vi "Discover Devices.vi"(8 "error in (no error)":errorcluster, 11 "Tree ref in":refnum<vi>) -> (0 "error out":errorcluster)   [LabVIEW 2022 SP3]
doc: "This example demonstrated how to create an openDAQ instance and detect devices.\nThen it goes through all detected devices and displays their name and manufacturer."
uses:
  <instrlib>/openDAQ/Public/Classes/IInstance/IInstance.lvclass
  C:/Program Files (x86)/National Instruments/LabVIEW 2022/instr.lib/openDAQ/Public/Classes/IDevice/IDevice.lvclass
  <instrlib>/openDAQ/Public/Classes/IInstanceBuilder/IInstanceBuilder.lvclass
  <instrlib>/openDAQ/Public/Classes/IDeviceInfo/IDeviceInfo.lvclass
  <instrlib>/openDAQ/Public/Classes/IDevice/IDevice.lvclass
panel:
  in  "MCL:available Devices":i32(listbox)
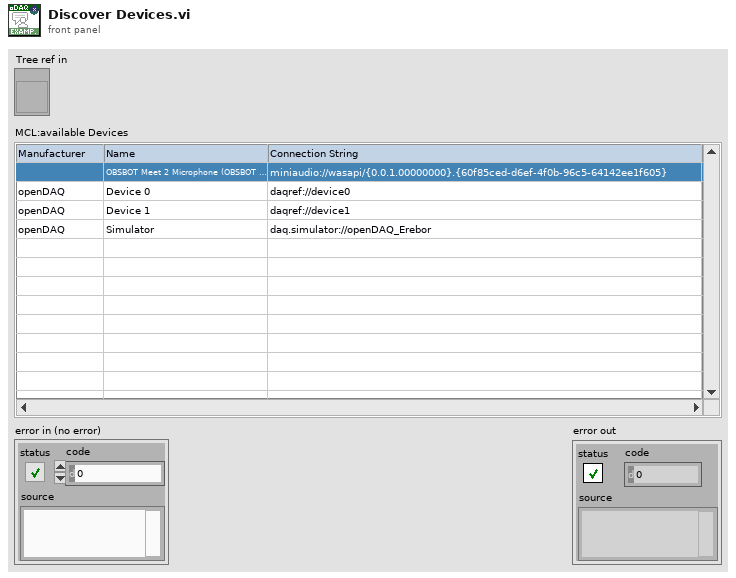
[diagram p1: front panel]
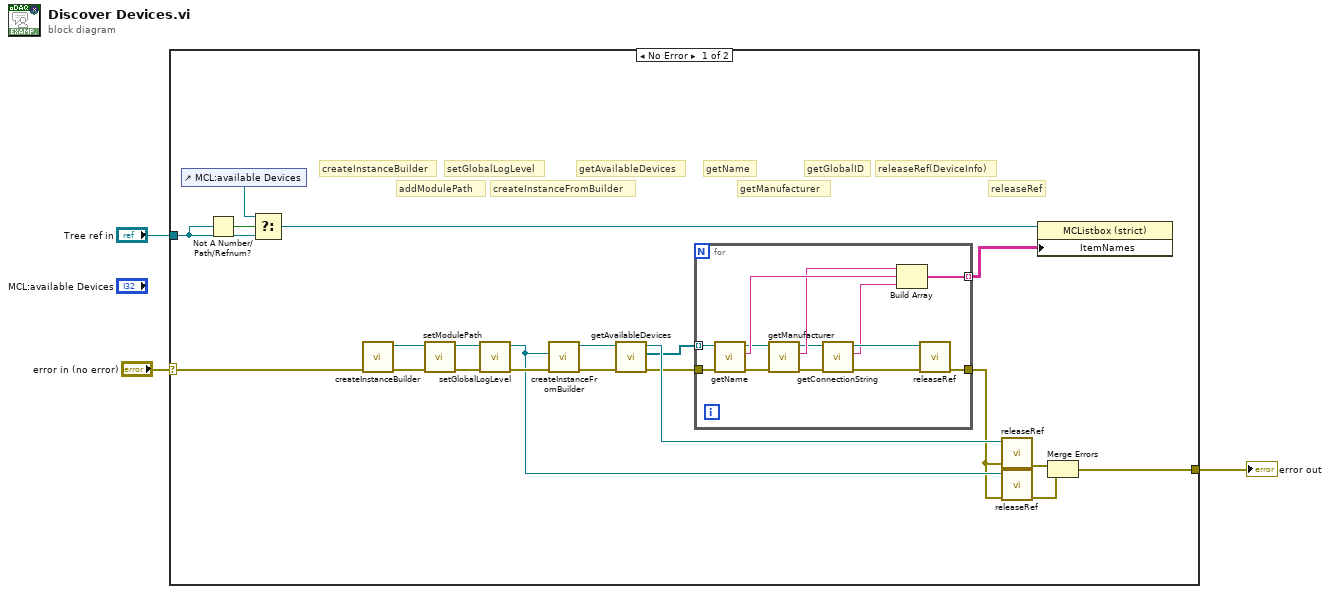
[diagram p0: block diagram]
diagram:
  n1 = case shown="No Error" "error in (no error)" {
    selector: "error in (no error)" -> [w23 w38]
    tunnel: [w24 w38] -> w3
    tunnel: "Tree ref in" -> [w6 _]
    frame No Error {
      # "getGlobalID"
      # "createInstanceFromBuilder"
      # "releaseRef(DeviceInfo)"
      # "getManufacturer"
      # "getName"
      # "releaseRef"
      # "getAvailableDevices"
      # "setGlobalLogLevel"
      # "addModulePath"
      # "createInstanceBuilder"
      n2 = control-ref of="MCL:available Devices"() -> (w5:refnum<vi>)
      n3 = Not A Number/Path/Refnum?(number/path/refnum=w6) -> (NaN/Path/Refnum?=w7:bool)
      n4 = Select(t=w5, s=w7, f=w6) -> (s? t:f=w4:refnum<vi>)
      n5 = call <instrlib>:"createInstanceBuilder.vi"("error in (no error)"=w23) -> ("error out"=w22:errorcluster, "IInstanceBuilder out"=w21:refnum<class "IInstanceBuilder.lvclass">)  [unwired: 9 in]
      n6 = call <instrlib>:"setModulePath.vi"("error in (no error)"=w22, "IInstanceBuilder in"=w21) -> ("error out"=w20:errorcluster, "IInstanceBuilder out"=w19:refnum<class "IInstanceBuilder.lvclass">)  [unwired: 8 in]
      n7 = call <instrlib>:"setGlobalLogLevel.vi"("error in (no error)"=w20, "IInstanceBuilder in"=w19) -> ("error out"=w18:errorcluster, "IInstanceBuilder out"=w12:refnum<class "IInstanceBuilder.lvclass">)  [unwired: 8 in]
      n8 = call <instrlib>:"createInstanceFromBuilder.vi"("error in (no error)"=w18, "IInstanceBuilder in"=w12) -> ("error out"=w17:errorcluster, "IInstance out"=w16:refnum<class "IInstance.lvclass">)  [unwired: 8 in]
      n9 = call <instrlib>:"getAvailableDevices.vi"("error in (no error)"=w17, "IDevice in"=w16) -> ("error out"=w13:errorcluster, "availableDeviceInfo out"=w14:refnum<class "IDeviceInfo.lvclass">[], "IDevice out"=w15:refnum<class "IInstance.lvclass">)  [unwired: 7 in]
      n10 = for {
        tunnel: [w37] -> w8 mode=indexing
        tunnel: w14 -> [w31] mode=indexing
        tunnel: w13 -> [w30]
        tunnel: [w32] -> w9
        n11 = call <instrlib>:"getName.vi"("error in (no error)"=w30, "IDeviceInfo in"=w31) -> ("error out"=w34:errorcluster, "Name out"=w36:string, "IDeviceInfo out"=w35:refnum<class "IDeviceInfo.lvclass">)  [unwired: 7 in]
        n12 = call <instrlib>:"getManufacturer.vi"("error in (no error)"=w34, "IDeviceInfo in"=w35) -> ("error out"=w28:errorcluster, "Manufacturer out"=w33:string, "IDeviceInfo out"=w29:refnum<class "IDeviceInfo.lvclass">)  [unwired: 7 in]
        n13 = call <instrlib>:"getConnectionString.vi"("error in (no error)"=w28, "IDeviceInfo in"=w29) -> ("error out"=w26:errorcluster, "ConntectionString out"=w25:string, "IDeviceInfo out"=w27:refnum<class "IDeviceInfo.lvclass">)  [unwired: 7 in]
        n14 = Build Array(w33, w36, w25) -> (w37:string[])
        n15 = call-dynamic "releaseRef.vi"("error in (no error)"=w26, "IBaseObject in"=w27) -> ("error out"=w32:errorcluster)  [unwired: 9 in]
      }
      n16 = call-dynamic "releaseRef.vi"("error in (no error)"=w9, "IBaseObject in"=w15) -> ("error out"=w11:errorcluster)  [unwired: 9 in]
      n17 = call-dynamic "releaseRef.vi"("error in (no error)"=w9, "IBaseObject in"=w12) -> ("error out"=w10:errorcluster)  [unwired: 9 in]
      n18 = property class="MCListbox (strict)"(reference=w4, "ItemNames"=w8) -> ()  [unwired: 1 in, 2 out]
      n19 = Merge Errors(w11, w10) -> (w24:errorcluster)
    }
    frame Error {
    }
  }
  "error out" <- w3
